vi "QSPARK_connectLaser.vi"(10 "password":string="QS_35", 11 "username":string="QSuser") -> (3 "client handle out":T1)   [LabVIEW 2024]
uses:
  <vilib>/httpClient/ClientHandle.ctl
  <vilib>/httpClient/LabVIEWHTTPClient.lvlib
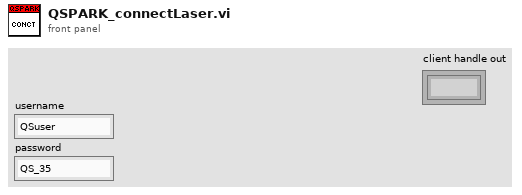
[diagram p1: front panel]
types:
  T1 = typedef "LabVIEWHTTPClient.lvlib/ClientHandle.ctl" = refnum<k1>
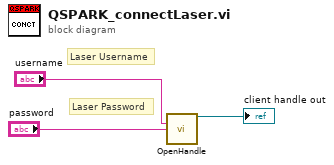
[diagram p0: block diagram]
diagram:
  # "Laser Password"
  # "Laser Username"
  n1 = call <vilib>:"OpenHandle.vi"("username"="username", "password"="password") -> ("client handle out"=→"client handle out":T1)  [unwired: 12 in, 1 out]
